vi "Calibrate.vi"(3 "Deviceindex":i32) -> (0 "Calib Error":bool, 1 "Status":string)   [LabVIEW 2011]
uses:
  MT Scan/SubVIs/hhlib.dll
panel:
  out "Returncode":i32
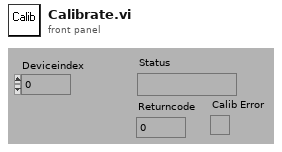
[diagram p1: front panel]
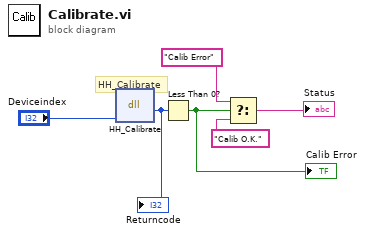
[diagram p0: block diagram]
diagram:
  # "HH_Calibrate"
  n1 = dll-call lib="C:/Users/Core-FCS/Desktop/AbelFCS/MT Scan/SubVIs/hhlib.dll" fn="HH_Calibrate"("devidx"="Deviceindex") -> (w4:i32)  [unwired: 4 in, 2 out]
  "Returncode" <- w4
  n2 = Less Than 0?(x=w4) -> (x < 0?=w2:bool)
  "Calib Error" <- w2
  n3 = Select(t="Calib Error", s=w2, f="Calib O.K.") -> (s? t:f=→"Status":string)
